vi "Read TCP Data.vi"(8 "error in (no error)":errorcluster caption="错误输入（无错误）", 11 "LS-H600-TCP Client 输入":refnum<class "LS-H600-TCP Client.lvclass">) -> (0 "error out":errorcluster caption="错误输出", 3 "LS-H600-TCP Client 输出":refnum<class "LS-H600-TCP Client.lvclass">)   [LabVIEW 2022 SP3, in "LS-H600-TCP Client.lvlib" / "LS-H600-TCP Client.lvclass"]
uses:
  LS-H600-TCP Client.lvclass
  C:/Program Files (x86)/National Instruments/LabVIEW 2022/vi.lib/ActorFramework/Actor/Actor.lvclass
  LS-H600-TCP Client.lvclass/LS-H600-TCP Client.ctl
  <vilib>/ActorFramework/Actor/Actor.lvclass/Actor.ctl
  <vilib>/ActorFramework/Message Enqueuer/Message Enqueuer.lvclass/Message Enqueuer.ctl
  <vilib>/ActorFramework/Message Enqueuer/Init from Existing Queue.vi
  <vilib>/ActorFramework/Message Enqueuer/Enqueue.vi
  C:/Program Files (x86)/National Instruments/LabVIEW 2022/vi.lib/ActorFramework/Message/Message.lvclass
  <vilib>/ActorFramework/Message Priority Queue/Priority Enqueue.vi
  <vilib>/ActorFramework/Message Enqueuer/Message Enqueuer.lvclass
  <vilib>/ActorFramework/Actor/Actor.lvclass
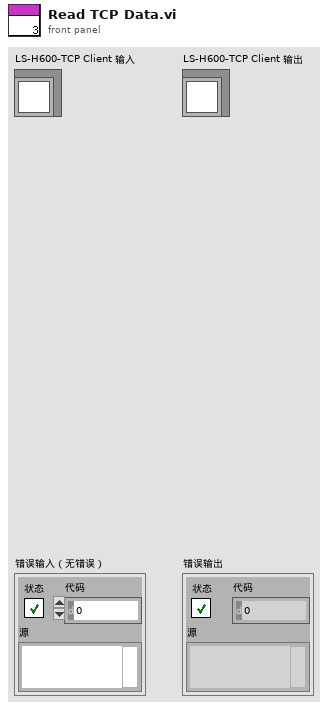
[diagram p1: front panel]
types:
  T1 = enum16{"Standard", "Buffered", "CRLF", "Immediate"}
  T2 = cluster{"时间":timestamp, "仪器水深":dbl, "水温":dbl, "流速":dbl, "过水面积":dbl, "瞬时流量":dbl, "累积流量":dbl, "剖面流速":dbl[]}
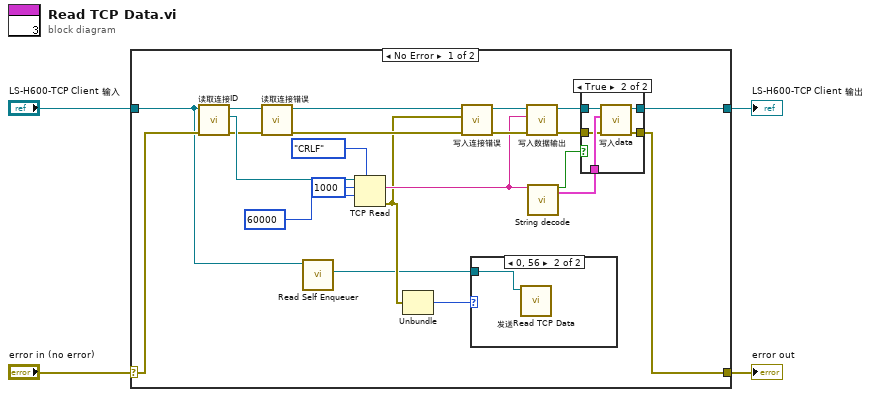
[diagram p0: block diagram]
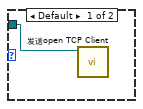
[diagram p2: hidden frame]
diagram:
  n1 = case shown="No Error" "error in (no error)" {
    selector: "error in (no error)" -> [w25 w37]
    tunnel: [w10 w37] -> w3
    tunnel: [w11 w36] -> w1
    tunnel: "LS-H600-TCP Client 输入" -> [w7 w36]
    frame No Error {
      n2 = call "读取连接ID.vi"("error in (no error)"=w25, "LS-H600-TCP Client输入"=w7) -> ("error out"=w23:errorcluster, "连接ID"=w26:refnum<k5>, "LS-H600-TCP Client输出"=w24:refnum<class "LS-H600-TCP Client.lvclass">)  [unwired: 7 in]
      n3 = call "读取连接错误.vi"("error in (no error)"=w23, "LS-H600-TCP Client输入"=w24) -> ("error out"=w18:errorcluster, "LS-H600-TCP Client输出"=w20:refnum<class "LS-H600-TCP Client.lvclass">)  [unwired: 7 in, 1 out]
      n4 = call <vilib>:"Read Self Enqueuer.vi"("Actor"=w7) -> ("Self Enqueuer"=w6:refnum<class "Message Enqueuer.lvclass">)  [unwired: 10 in]
      n5 = TCP Read(connection ID=w26, bytes to read=1000 ("读取的字节"), 7:T1."CRLF" ("模式（标准）"), 9:60000 ("超时毫秒(25000)")) -> (data out=w16:string, error out=w9:errorcluster)  [unwired: 1 in, 1 out]
      n6 = Unbundle(w9) -> ("code"=w8:i32)  [unwired: 2 out]
      n7 = call "写入连接错误.vi"("error in (no error)"=w18, "连接错误"=w9, "LS-H600-TCP Client输入"=w20) -> ("error out"=w17:errorcluster, "LS-H600-TCP Client输出"=w19:refnum<class "LS-H600-TCP Client.lvclass">)  [unwired: 7 in]
      n8 = case shown="0, 56" w8 {
        tunnel: w6 -> [w27 w28]
        frame Default {
          n9 = call "发送open TCP Client.vi"("Message Enqueuer"=w27) -> ()  [unwired: 9 in, 2 out]
        }
        frame 0, 56 {
          n10 = call "发送Read TCP Data.vi"("Message Enqueuer"=w28) -> ()  [unwired: 9 in, 2 out]
        }
      }
      n11 = call "写入数据输出.vi"("error in (no error)"=w17, "数据输出"=w16, "LS-H600-TCP Client输入"=w19) -> ("error out"=w12:errorcluster, "LS-H600-TCP Client输出"=w15:refnum<class "LS-H600-TCP Client.lvclass">)  [unwired: 7 in]
      n12 = call "String decode.vi"("INPUT String"=w16) -> ("new data?"=w13:bool, "data"=w14:T2)  [unwired: 17 in]
      n13 = case shown="True" w13 {
        tunnel: w15 -> [w30 w35]
        tunnel: w14 -> [_ w34]
        tunnel: w12 -> [w29 w33]
        tunnel: [w30 w32] -> w11
        tunnel: [w29 w31] -> w10
        frame False {
        }
        frame True {
          n14 = call "写入data.vi"("error in (no error)"=w33, "data"=w34, "LS-H600-TCP Client输入"=w35) -> ("error out"=w31:errorcluster, "LS-H600-TCP Client输出"=w32:refnum<class "LS-H600-TCP Client.lvclass">)  [unwired: 7 in]
        }
      }
    }
    frame Error {
    }
  }
  "error out" <- w3
  "LS-H600-TCP Client 输出" <- w1
